vi "Run.vi"(8 "error in (no error)":errorcluster caption="entrée d'erreur (pas d'erreur)", 11 "California_housing.lvclass":refnum<class "California_housing.lvclass">) -> (0 "error out":errorcluster caption="sortie d'erreur", 2 "Data":T1, 3 "California_housing.lvclass":refnum<class "California_housing.lvclass">)   [LabVIEW 2020, in "California_housing.lvclass"]
doc: "Returns :\n\n- data : ndarray, shape (20640, 8)\nEach row corresponding to the 8 feature values in order. If as_frame is True, data is a pandas object.\n\n\n- target : numpy array of shape (20640,)\nEach value corresponds to the average house value in units of 100,000. If as_frame is True, target is a pandas object."
uses:
  California_housing.lvclass
  California_housing.lvclass/California_housing.ctl
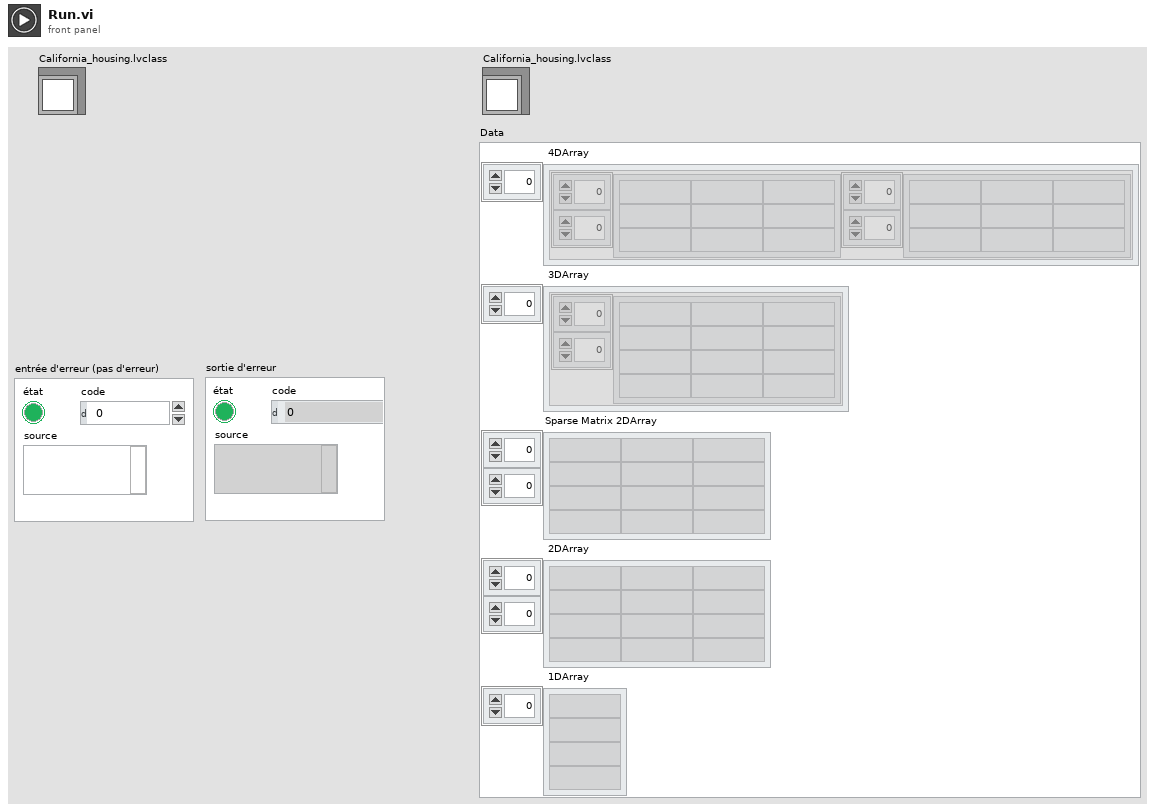
[diagram p1: front panel]
types:
  T1 = cluster{" 4DArray":cluster{"1":string[][], "2":string[][]}[], " 3DArray":cluster{"Tableau":string[][]}[], "Sparse Matrix 2DArray":string[][], " 2DArray":string[][], " 1DArray":string[]}
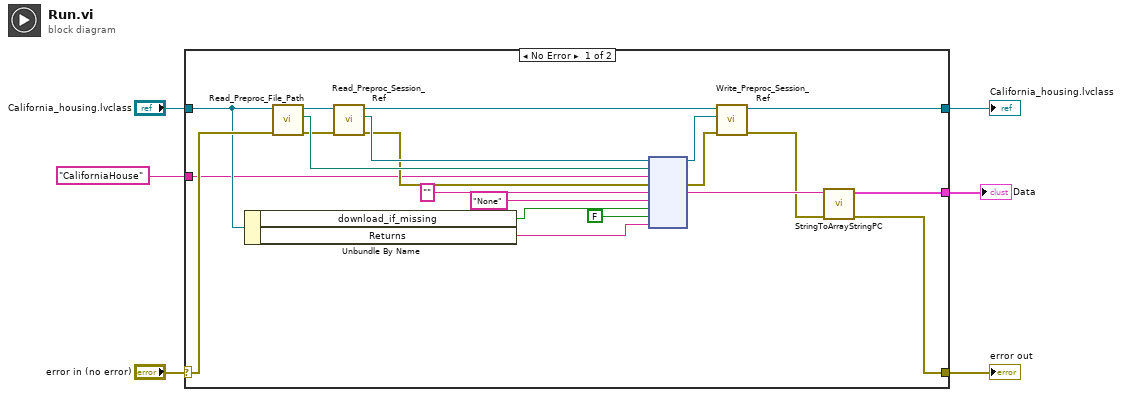
[diagram p0: block diagram]
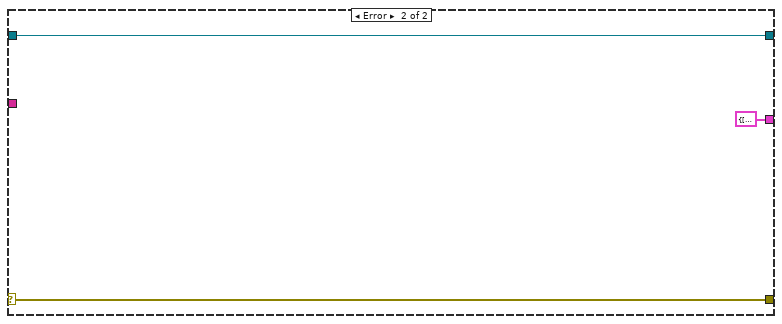
[diagram p2: hidden frame]
diagram:
  n1 = case shown="No Error" "error in (no error)" {
    selector: "error in (no error)" -> [w18 w30]
    tunnel: [w8 w30] -> w5
    tunnel: [w11 w29] -> w3
    tunnel: "California_housing.lvclass" -> [w17 w29]
    tunnel: "CaliforniaHouse" -> [w16 _]
    tunnel: [w7 T1 {" 4DArray"=[], " 3DArray"=[], "Sparse Matrix 2DArray"=[], " 2DArray"=[], " 1DArray"=[]} ("Data")] -> w1
    frame No Error {
      n2 = Unbundle By Name(w17) -> ("download_if_missing"=w15:bool, "Returns"=w12:string)
      n3 = call-dynamic "Read_Preproc_File_Path.vi"("error in (no error)"=w18, "Python in"=w17) -> ("error out"=w22:errorcluster, "File_Path"=w25:path, "Python out"=w27:refnum<class "California_housing.lvclass">)  [unwired: 7 in]
      n4 = call-dynamic "Read_Preproc_Session_Ref.vi"("error in (no error)"=w22, "Python in"=w27) -> ("error out"=w23:errorcluster, "Session_ref"=w24:refnum<k35>, "Python out"=w26:refnum<class "California_housing.lvclass">)  [unwired: 7 in]
      n5 = node(w24, w25, w16, w23, "", "None", w15, FALSE, w12) -> (w19:refnum<k35>, w21:errorcluster, w10:string)  [unwired: 4 in, 2 out]
      n6 = call-dynamic "Write_Preproc_Session_Ref.vi"("error in (no error)"=w21, "Session_ref"=w19, "Python in"=w26) -> ("error out"=w9:errorcluster, "Python out"=w11:refnum<class "California_housing.lvclass">)  [unwired: 7 in]
      n7 = call "StringToArrayStringPC.vi"("sortie d'erreur"=w9, "Return value"=w10) -> ("sortie d'erreur"=w8:errorcluster, "Data"=w7:T1)  [unwired: 8 in]
    }
    frame Error {
    }
  }
  "error out" <- w5
  "California_housing.lvclass" <- w3
  "Data" <- w1
